vi "GetAllLVProjects.vi"(8 "error in (no error)":errorcluster) -> (0 "error out":errorcluster, 2 "LVProj names":string[](array[string]), 3 "LVProj paths":path[](array[path]))   [LabVIEW 2019, in "Hawkeye.lvlib"]
uses:
  Hawkeye.lvlib
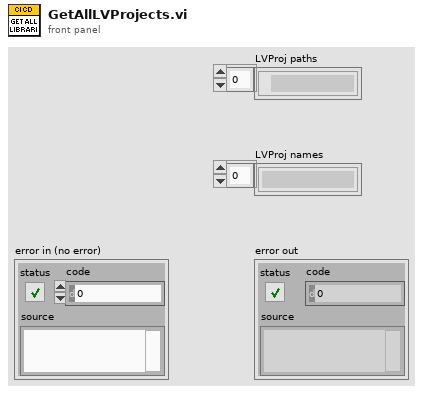
[diagram p1: front panel]
types:
  T1 = typedef "Hawkeye.lvlib/CICDPathConfigs.ctl" = cluster{"GlobalIncludePaths":path[], "GlobalExcludePaths":path[], "BuildSpecsIncludePaths":path[], "ActualDepsIncludePaths":path[], "WorkspacePath":path, "SourceFolderPaths":path[], "ChangedFilesLogpaths":map{string, path}}
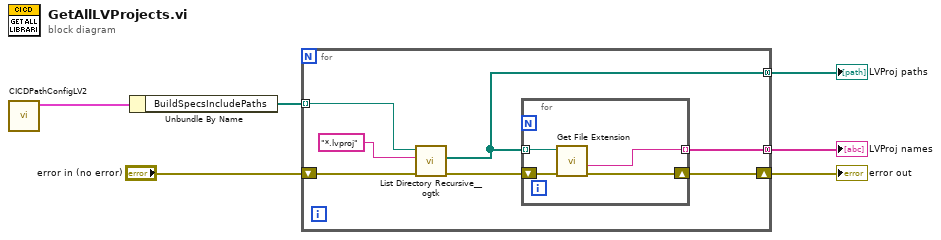
[diagram p0: block diagram]
diagram:
  n1 = call "CICDPathConfigLV2.vi"() -> ("CICD Path Config Out"=w2:T1)  [unwired: 11 in]
  n2 = Unbundle By Name(w2) -> ("BuildSpecsIncludePaths"=w5:path[])
  n3 = for {
    tunnel: [w10] -> w3 mode=concatenating
    shift-right: [w7] -> w4
    shift-left: "error in (no error)" -> [w13]
    tunnel: w5 -> [w11] mode=indexing
    tunnel: [w9] -> w1 mode=concatenating
    n4 = call <userlib>:"List Directory Recursive__ogtk.vi"("error in (no error)"=w13, "pattern"="*.lvproj", "Path"=w11) -> ("error out"=w8:errorcluster, "file paths"=w10:path[])  [unwired: 5 in, 2 out]
    n5 = for {
      tunnel: w10 -> [w17] mode=indexing
      tunnel: [w16] -> w9 mode=indexing
      shift-right: [w14] -> w7
      shift-left: w8 -> [w15]
      n6 = call <vilib>:"Get File Extension.vi"("error in (no error)"=w15, "file"=w17) -> ("error out"=w14:errorcluster, "filename without extension"=w16:string)  [unwired: 5 in, 3 out]
    }
  }
  "error out" <- w4
  "LVProj paths" <- w3
  "LVProj names" <- w1
